vi "Set General Setup.vi"(8 "error in (no error)":errorcluster, 9 "General Setup":T2={"Export Path"=path "C:/Glass", "level"=0.8, "Time Gap"=20.0}, 11 "Map":T1) -> (0 "error out":errorcluster, 3 "Map Out":T1)   [LabVIEW 2015, in "ConfigHelper.lvlib"]
uses:
  ConfigHelper.lvlib
  Control_General Setup (Path).ctl
  <vilib>/addons/PointValueMap/controls/PointMap.ctl
  <vilib>/addons/PointValueMap/subVIs/Point_Write_variant.vi
  <vilib>/addons/PointValueMap/PointValueMap.lvlib
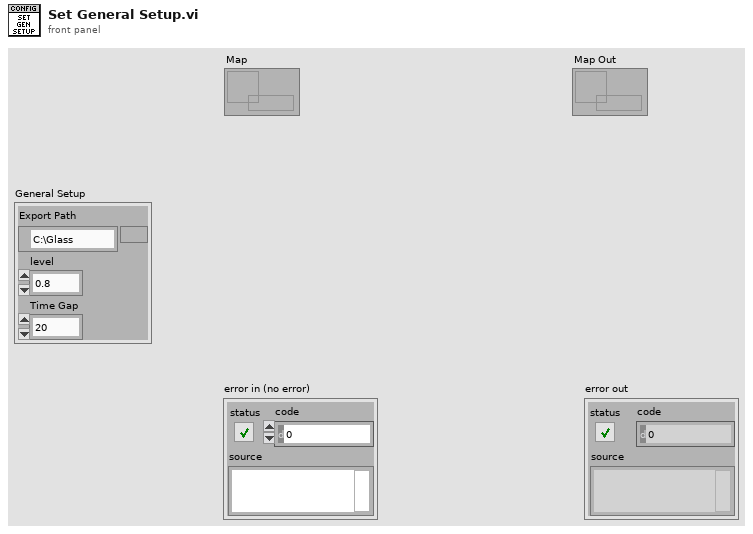
[diagram p1: front panel]
types:
  T1 = typedef "PointValueMap.lvlib/PointMap.ctl" = refnum<data-value>
  T2 = typedef "ConfigHelper.lvlib/Control_General Setup (Path).ctl" = cluster{"Export Path":path, "level":dbl, "Time Gap":dbl}
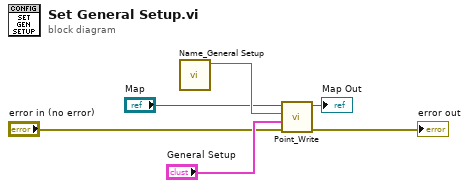
[diagram p0: block diagram]
diagram:
  n1 = call "Name_General Setup.vi"() -> ("Name"=w6:string)  [unwired: 11 in]
  n2 = call-poly <vilib>:"Point_Write.vi"("Error In"="error in (no error)", "Value"="General Setup", "Tag"=w6, "Map"="Map") -> ("Error Out"=→"error out":errorcluster, "Map Out"=→"Map Out":T1)  [unwired: 6 in]
